vi "FdxCmdTxSAPWriteCvi.vi"(4 "ByteCount":i32=-1, 6 "IpDst":u32, 7 "UdpDst":u32, 8 "error in":errorcluster, 9 "Data":u8[](array[numeric]), 10 "UdpHandle":u32, 11 "InstrumentHandle":u32) -> (0 "error out":errorcluster, 1 "BytesWritten":u32, 2 "UdpHandleOut":u32, 3 "InstrumentHandle":u32)   [LabVIEW 2020, in "AIM664LV.lvlib"]
doc: "This function is used to write a pure message to a SAP type port. The port must be an SAP type Transmit port.\nThis function can be used if the transmitter is running or not running."
uses:
  AIM664LV.lvlib
  AFDX_LibraryAdmin/FdxGlobalDllPath.vi
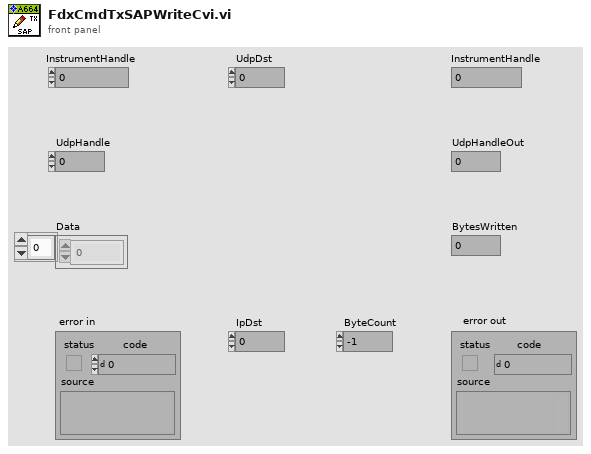
[diagram p1: front panel]
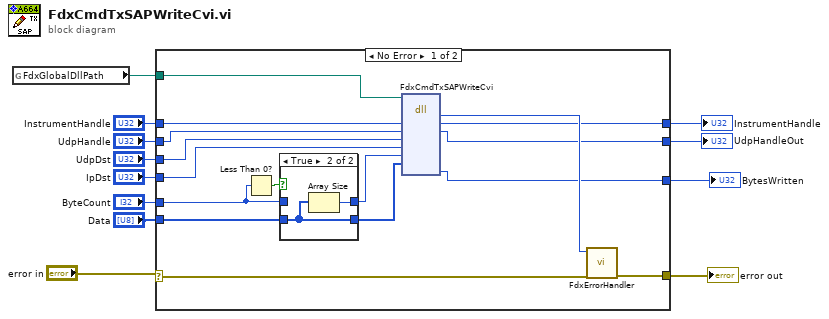
[diagram p0: block diagram]
diagram:
  n1 = global read "FdxGlobalDllPath.vi" "FdxGlobalDllPath"() -> (w10:path)
  n2 = case shown="No Error" "error in" {
    selector: "error in" -> [w27 w35]
    tunnel: [w28 w35] -> w12
    tunnel: w10 -> [w25 _]
    tunnel: "InstrumentHandle" -> [w23 w34]
    tunnel: [w24 w34] -> w8
    tunnel: "UdpHandle" -> [w22 w33]
    tunnel: [w21 w33] -> w6
    tunnel: "UdpDst" -> [w20 _]
    tunnel: "IpDst" -> [w19 _]
    tunnel: "ByteCount" -> [w17 _]
    tunnel: "Data" -> [w16 _]
    tunnel: [w13 _] -> w1
    frame No Error {
      n3 = Less Than 0?(x=w17) -> (x < 0?=w18:bool)
      n4 = case shown="True" w18 {
        tunnel: w16 -> [w29 w31]
        tunnel: w17 -> [w30 _]
        tunnel: [w30 w32] -> w14
        tunnel: [w29 w31] -> w15
        frame False {
        }
        frame True {
          n5 = Array Size(array=w31) -> (size(s)=w32:i32)
        }
      }
      n6 = dll-call lib="aim_fdx.19.dll" fn="FdxCmdTxSAPWriteCvi"(path in=w25, "InstrumentHandle"=w23, "UdpHandle"=w22, "UdpDst"=w20, "IpDst"=w19, "ByteCount"=w14, "Data"=w15) -> ("status"=w26:i32, "InstrumentHandle"=w24:u32, "UdpHandle"=w21:u32, "BytesWritten"=w13:u32)  [unwired: 6 in, 3 out]
      n7 = call "FdxErrorHandler.vi"("error in"=w27, "AIM Error"=w26) -> ("error out"=w28:errorcluster)  [unwired: 9 in]
    }
    frame Error {
    }
  }
  "error out" <- w12
  "InstrumentHandle" <- w8
  "UdpHandleOut" <- w6
  "BytesWritten" <- w1
